vi "Test8.vi"() -> ()   [LabVIEW 2010]
uses:
  <vilib>/MDSplus/Library/MDSplus.lvlib
  <vilib>/MDSplus/Classes/Data_Class/Data.lvclass
  <vilib>/MDSplus/Classes/Data_Class/TreeNode_Class/TreeNode.lvclass
panel:
  in  "SGL array in":sgl[](array[numeric])=[1.11, 2.22, 3.33, 4.44]
  out "SGL out 2":sgl
  out "SGL out":sgl
  out "SGL array out":sgl[](array[numeric])
  in  "Value":sgl=6.666
  in  "Path":string=":NUMX"
  in  "Mode":string="EDIT"
  in  "Shot":i32=-1
  in  "Name":string="my_tree"
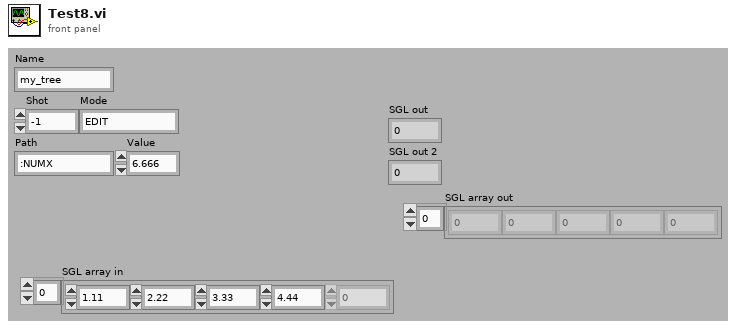
[diagram p1: front panel]
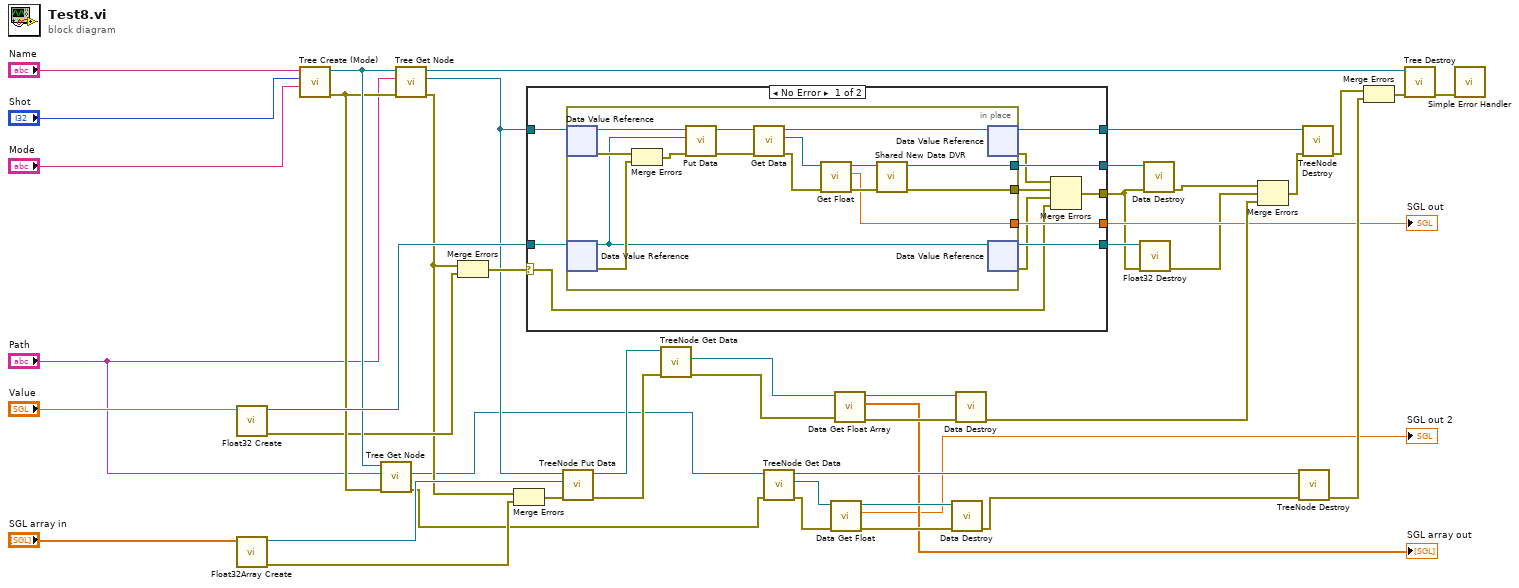
[diagram p0: block diagram]
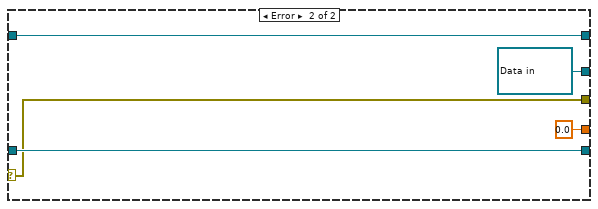
[diagram p2: hidden frame]
diagram:
  n1 = call <vilib>:"Float32 Create.vi"("SGL in"="Value") -> ("error out"=w16:errorcluster, "Float32 DVR out"=w40:refnum<data-value>)  [unwired: 9 in]
  n2 = call <vilib>:"Float32Array Create.vi"("SGL array in"="SGL array in") -> ("error out"=w3:errorcluster, "Float32Array DVR out"=w24:refnum<data-value>)  [unwired: 9 in]
  n3 = call <vilib>:"Tree Create (Mode).vi"("Mode"="Mode", "Shot"="Shot", "Name"="Name") -> ("error out"=w32:errorcluster, "Tree DVR out"=w33:refnum<data-value>)  [unwired: 7 in]
  n4 = call <vilib>:"Tree Get Node.vi"("error in (no error)"=w32, "Path"="Path", "Tree DVR in"=w33) -> ("error out"=w1:errorcluster, "TreeNode DVR out"=w4:refnum<data-value>)  [unwired: 5 in, 1 out]
  n5 = call <vilib>:"Tree Get Node.vi"("error in (no error)"=w32, "Path"="Path", "Tree DVR in"=w33) -> ("error out"=w9:errorcluster, "TreeNode DVR out"=w10:refnum<data-value>, "Tree DVR out"=w41:refnum<data-value>)  [unwired: 5 in]
  n6 = Merge Errors(w9, w16) -> (w17:errorcluster)
  n7 = Merge Errors(w9, w3) -> (w2:errorcluster)
  n8 = case shown="No Error" w17 {
    selector: w17 -> [w47 w75]
    tunnel: [w54 w76] -> w42
    tunnel: w40 -> [w55 w77]
    tunnel: w10 -> [w56 w76]
    tunnel: [w51 w75] -> w13
    tunnel: [w57 sgl 0.0 ("SGL out")] -> w23
    tunnel: [w53 w77] -> w14
    tunnel: [w52 refnum<data-value> refnum ("Data DVR out")] -> w15
    frame No Error {
      n9 = in-place {
        in-place-border: [w58] -> w50
        in-place-border: [w69] -> w57
        in-place-border: [w62] -> w52
        n10 = in-place-dvr #1(w56) -> (w68:refnum<class "TreeNode.lvclass">, w67:errorcluster)
        n11 = in-place-dvr #2(w55) -> (w59:refnum<class "Float32.lvclass">, w66:errorcluster)
        n12 = Merge Errors(w67, w66) -> (w65:errorcluster)
        n13 = call-dynamic "Put Data.vi"("error in (no error)"=w65, "Data in"=w59, "TreeNode in"=w68) -> ("error out"=w60:errorcluster, "TreeNode out"=w64:refnum<class "TreeNode.lvclass">)  [unwired: 7 in]
        n14 = call-dynamic "Get Data.vi"("error in (no error)"=w60, "TreeNode in"=w64) -> ("error out"=w71:errorcluster, "Data out"=w72:refnum<class "Data.lvclass">, "TreeNode out"=w61:refnum<class "TreeNode.lvclass">)  [unwired: 7 in]
        n15 = call-dynamic "Get Float.vi"("error in (no error)"=w71, "Data in"=w72) -> ("error out"=w70:errorcluster, "SGL out"=w69:sgl, "Data out"=w63:refnum<class "Data.lvclass">)  [unwired: 7 in]
        n16 = call <vilib>:"Shared New Data DVR.vi"("error in (no error)"=w70, "Data in"=w63) -> ("error out"=w58:errorcluster, "Data DVR out"=w62:refnum<data-value>)  [unwired: 8 in]
        n17 = in-place-dvr #1(w61) -> (w54:refnum<data-value>, w49:errorcluster)
        n18 = in-place-dvr #2(w59) -> (w53:refnum<data-value>, w48:errorcluster)
      }
      n19 = Merge Errors(w49, w50, w48, w47) -> (w51:errorcluster)
    }
    frame Error {
    }
  }
  "SGL out" <- w23
  n20 = call <vilib>:"TreeNode Put Data.vi"("error in (no error)"=w2, "Data DVR in"=w24, "TreeNode DVR in"=w10) -> ("error out"=w6:errorcluster, "TreeNode DVR out"=w5:refnum<data-value>)  [unwired: 6 in]
  n21 = call <vilib>:"TreeNode Get Data.vi"("error in (no error)"=w6, "TreeNode DVR in"=w5) -> ("error out"=w21:errorcluster, "Data DVR out"=w20:refnum<data-value>)  [unwired: 6 in, 1 out]
  n22 = call <vilib>:"TreeNode Get Data.vi"("error in (no error)"=w1, "TreeNode DVR in"=w4) -> ("error out"=w34:errorcluster, "Data DVR out"=w22:refnum<data-value>, "TreeNode DVR out"=w37:refnum<data-value>)  [unwired: 6 in]
  n23 = call <vilib>:"Data Get Float.vi"("error in (no error)"=w34, "Data DVR in"=w22) -> ("error out"=w36:errorcluster, "SGL out"=→"SGL out 2":sgl, "Data DVR out"=w35:refnum<data-value>)  [unwired: 6 in]
  n24 = call <vilib>:"Data Get Float Array.vi"("error in (no error)"=w21, "Data DVR in"=w20) -> ("error out"=w27:errorcluster, "SGL array out"=→"SGL array out":sgl[], "Data DVR out"=w28:refnum<data-value>)  [unwired: 5 in, 1 out]
  n25 = call <vilib>:"Data Destroy.vi"("error in (no error)"=w36, "Data DVR in"=w35) -> ("error out"=w38:errorcluster)  [unwired: 8 in]
  n26 = call <vilib>:"Data Destroy.vi"("error in (no error)"=w27, "Data DVR in"=w28) -> ("error out"=w26:errorcluster)  [unwired: 8 in]
  n27 = call <vilib>:"Float32 Destroy.vi"("error in (no error)"=w13, "Scalar DVR in"=w14) -> ("error out"=w11:errorcluster)  [unwired: 8 in]
  n28 = call <vilib>:"Data Destroy.vi"("error in (no error)"=w13, "Data DVR in"=w15) -> ("error out"=w12:errorcluster)  [unwired: 8 in]
  n29 = Merge Errors(w12, w11, w26) -> (w25:errorcluster)
  n30 = call <vilib>:"TreeNode Destroy.vi"("error in (no error)"=w38, "TreeNode DVR in"=w37) -> ("error out"=w31:errorcluster)  [unwired: 8 in]
  n31 = call <vilib>:"TreeNode Destroy.vi"("error in (no error)"=w25, "TreeNode DVR in"=w42) -> ("error out"=w30:errorcluster)  [unwired: 8 in]
  n32 = Merge Errors(w30, w31) -> (w29:errorcluster)
  n33 = call <vilib>:"Tree Destroy.vi"("error in (no error)"=w29, "Tree DVR in"=w41) -> ("error out"=w39:errorcluster)  [unwired: 8 in]
  n34 = call <vilib>:"Simple Error Handler.vi"("error in (no error)"=w39) -> ()  [unwired: 4 in, 5 out]
